vi "scaleatoms.vi"(1 "Atoms Image":dbl[][](array[numeric])=[[0.0, 0.0, 0.0, 0.0, 0.0, 0.0, 0.0, 0.0, 0.0, 0.0, 0.0, 1.0], [0.0, 1.0, 0.0, 0.0, 0.0, 0.0, 0.0, 0.0, 0.0, 0.0, 2.0, 0.0], [0.0, 0.0, 2.0, 0.0, 0.0, 0.0, 0.0, 0.0, 0.0, 3.0, 0.0, 0.0], [0.0, 0.0, 0.0, 3.0, 0.0, 0.0, 0.0, 0.0, 4.0, 0.0, 0.0, 0.0], [0.0, 0.0, 0.0, 0.0, 4.0, 0.0, 0.0, 5.0, 0.0, 0.0, 0.0, 0.0], [0.0, 0.0, 0.0, 0.0, 0.0, 5.0, 6.0, 0.0, 0.0, 0.0, 0.0, 0.0], [0.0, 0.0, 0.0, 0.0, 0.0, 7.0, 6.0, 0.0, 0.0, 0.0, 0.0, 0.0], [3.0, 0.0, 0.0, 0.0, 8.0, 0.0, 0.0, 7.0, 0.0, 0.0, 0.0, 0.0], [0.0, 2.0, 0.0, 9.0, 0.0, 0.0, 0.0, 0.0, 8.0, 0.0, 8.0, 7.0], [3.0, 0.0, 1.0, 0.0, 0.0, 0.0, 0.0, 0.0, 0.0, 9.0, 0.0, 2.0]] format="%.2f", 2 "Scale atoms to bg level?":bool, 3 "Background Image":dbl[][](array[numeric])=[[0.0, 0.0, 0.0, 0.0, 0.0, 0.0, 0.0, 0.0, 0.0, 0.0, 0.0, 1.0], [0.0, 1.0, 0.0, 0.0, 0.0, 0.0, 0.0, 0.0, 0.0, 0.0, 2.0, 0.0], [0.0, 0.0, 2.0, 0.0, 0.0, 0.0, 0.0, 0.0, 0.0, 3.0, 0.0, 0.0], [0.0, 0.0, 0.0, 3.0, 0.0, 0.0, 0.0, 0.0, 4.0, 0.0, 0.0, 0.0], [0.0, 0.0, 0.0, 0.0, 4.0, 0.0, 0.0, 5.0, 0.0, 0.0, 0.0, 0.0], [0.0, 0.0, 0.0, 0.0, 0.0, 5.0, 6.0, 0.0, 0.0, 0.0, 0.0, 0.0], [0.0, 0.0, 0.0, 0.0, 0.0, 7.0, 6.0, 0.0, 0.0, 0.0, 0.0, 0.0], [3.0, 0.0, 0.0, 0.0, 8.0, 0.0, 0.0, 7.0, 0.0, 0.0, 0.0, 0.0], [0.0, 2.0, 0.0, 9.0, 0.0, 0.0, 0.0, 0.0, 8.0, 0.0, 8.0, 7.0], [3.0, 0.0, 1.0, 0.0, 0.0, 0.0, 0.0, 0.0, 0.0, 9.0, 0.0, 2.0]] format="%.2f") -> (0 "Atoms Scaled":dbl[][](array[numeric]))   [LabVIEW 2013]
panel:
  out "Atoms\n image":dbl[][](graph)
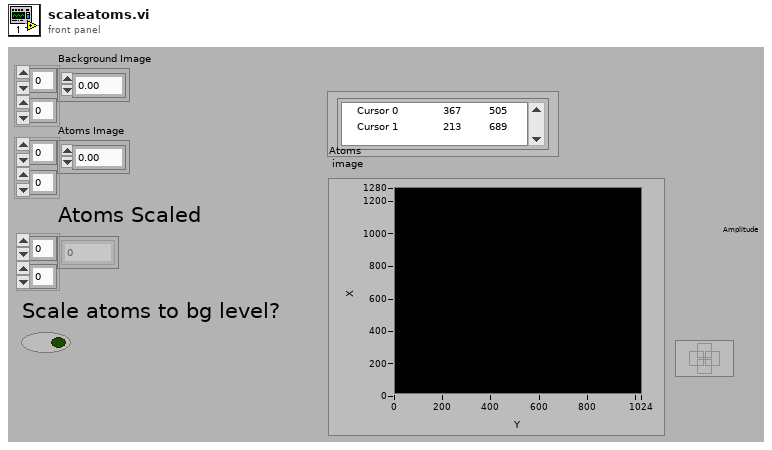
[diagram p1: front panel]
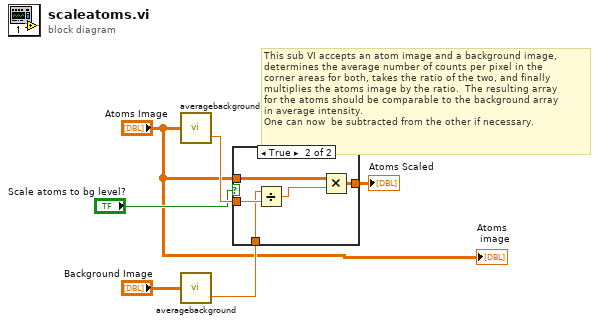
[diagram p0: block diagram]
diagram:
  # "This sub VI accepts an atom image and a background image, \ndetermines the average number of counts per pixel in the \ncorner areas for both, takes the ratio of the two, and finally \nmultiplies the atoms image by the ratio.  The resulting array \nfor the atoms should be comparable to the background array \nin average intensity.\nOne can now  be subtracted from the other if necessary."
  n1 = call "averagebackground.vi"("Input Array"="Atoms Image") -> ("average # of counts in corner areas"=w6:dbl)  [unwired: 1 out]
  n2 = call "averagebackground.vi"("Input Array"="Background Image") -> ("average # of counts in corner areas"=w5:dbl)  [unwired: 1 out]
  n3 = case shown="True" "Scale atoms to bg level?" {
    tunnel: w6 -> [_ w12]
    tunnel: w5 -> [_ w11]
    tunnel: "Atoms Image" -> [w7 w10]
    tunnel: [w7 w8] -> w3
    frame False {
    }
    frame True {
      n4 = Divide(x=w11, y=w12) -> (x/y=w9:dbl)
      n5 = Multiply(x=w10, y=w9) -> (x*y=w8:dbl[][])
    }
  }
  "Atoms Scaled" <- w3
  "Atoms\n image" <- "Atoms Image"
